vi "Plugin.Create.vi"(5 "Debug Flags":refnum<class "Debug Flags.lvclass">, 7 "transceiver count":i32, 8 "error in (no error)":errorcluster, 9 "component classes":refnum<class>[](array[class]), 10 "Plugin Configuration":refnum<class "Plugin Configuration.lvclass">, 11 "Transfer Groups":refnum<class "Transfer Group.lvclass">[](array[class])) -> (0 "error out":errorcluster, 2 "Transceiver":refnum<class "Transceiver.lvclass">, 3 "Plugin out":refnum<class "Plugin.lvclass">)   [LabVIEW 2017, in "DSF Core.lvlib" / "Plugin.lvclass"]
uses:
  Plugin.lvclass
  Transfer/Transfer Group.lvclass
  Debug/Debug Flags.lvclass
  Shared/Classes/Plugin/Plugin Configuration.lvclass
  C:/Git/DSF/dsf core/Source/Shared/Classes/Configuration/Configuration.lvclass
  Transceiver/Transceiver.lvclass
  Shared/Classes/Configuration/Configuration.lvclass/Configuration.ctl
  Shared/Classes/Plugin/Plugin Configuration.lvclass/Plugin Configuration.ctl
  Plugin.lvclass/Plugin.ctl
  Timing/Timing.lvclass
  Shared/Classes/Configuration/Configuration.lvclass
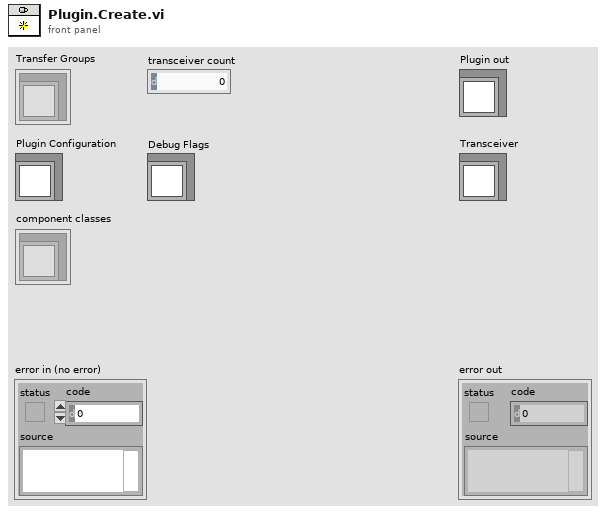
[diagram p1: front panel]
types:
  T1 = typedef "DSF Core.lvlib/DSF Timing Info.ctl" = cluster{"priority":u64, "decimation":u64, "offset":u64}
  T2 = typedef "DSF Core.lvlib/DSF Settings Info.ctl" = cluster{"key":string, "value":string}[]
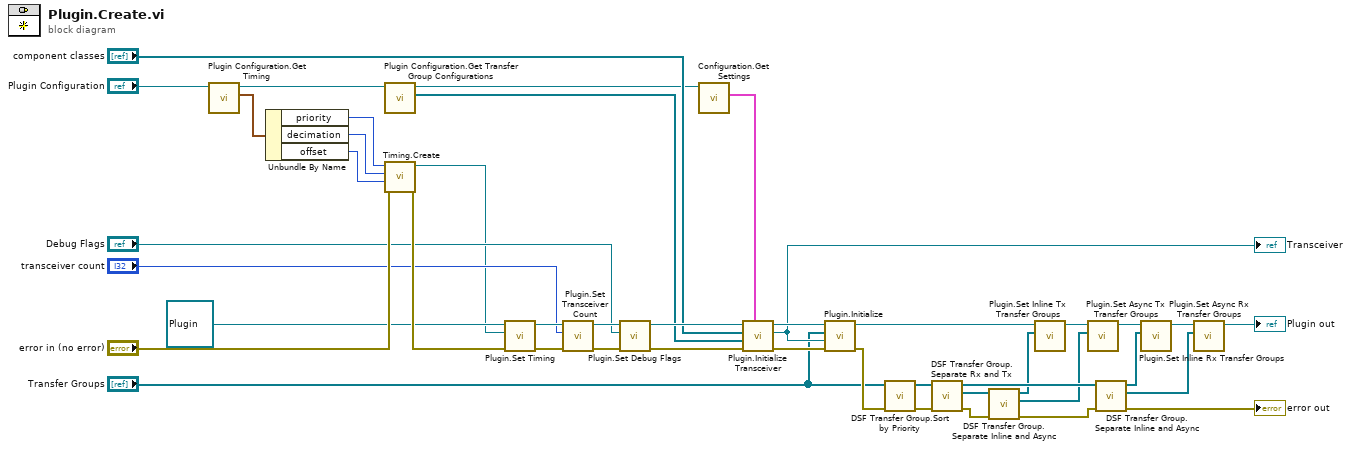
[diagram p0: block diagram]
diagram:
  n1 = call "Plugin Configuration.Get Timing.vi"("Plugin Configuration in"="Plugin Configuration") -> ("cycle timing"=w16:T1, "Plugin Configuration out"=w11:refnum<class "Plugin Configuration.lvclass">)  [unwired: 9 in]
  n2 = Unbundle By Name(w16) -> ("priority"=w13:u64, "decimation"=w14:u64, "offset"=w15:u64)
  n3 = call "Plugin Configuration.Get Transfer Group Configurations.vi"("Plugin Configuration in"=w11) -> ("Transfer Group Configurations"=w6:refnum<class "Transfer Group Configuration.lvclass">[], "Plugin Configuration out"=w2:refnum<class "Plugin Configuration.lvclass">)  [unwired: 9 in]
  n4 = call "Timing.Create.vi"("error in (no error)"="error in (no error)", "Offset"=w15, "Decimation"=w14, "Priority"=w13) -> ("error out"=w39:errorcluster, "Timing"=w10:refnum<class "Timing.lvclass">)  [unwired: 6 in]
  n5 = call "Plugin.Set Timing.vi"("Timing"=w10, "Plugin in"=refnum<class "Plugin.lvclass"> refnum) -> ("Plugin out"=w36:refnum<class "Plugin.lvclass">)  [unwired: 9 in]
  n6 = call "Plugin.Set Transceiver Count.vi"("transceiver count"="transceiver count", "Plugin in"=w36) -> ("Plugin out"=w23:refnum<class "Plugin.lvclass">)  [unwired: 9 in]
  n7 = call "Plugin.Set Debug Flags.vi"("Debug Flags"="Debug Flags", "Plugin in"=w23) -> ("Plugin out"=w9:refnum<class "Plugin.lvclass">)  [unwired: 9 in]
  n8 = call "Configuration.Get Settings.vi"("Configuration in"=w2) -> ("settings"=w1:T2)  [unwired: 9 in, 1 out]
  n9 = call "Plugin.Initialize Transceiver.vi"("transceiver settings"=w1, "error in (no error)"=w39, "Transfer Groups Configurations"=w6, "component classes"="component classes", "Plugin in"=w9) -> ("error out"=w4:errorcluster, "Transceiver"=w5:refnum<class "Transceiver.lvclass">, "Plugin out"=w8:refnum<class "Plugin.lvclass">)  [unwired: 4 in]
  "Transceiver" <- w5
  n10 = call "Plugin.Initialize.vi"("error in (no error)"=w4, "Transceiver"=w5, "Transfer Groups"="Transfer Groups", "Plugin in"=w8) -> ("error out"=w19:errorcluster, "Plugin out"=w21:refnum<class "Plugin.lvclass">)  [unwired: 6 in]
  n11 = call "DSF Transfer Group.Sort by Priority.vi"("error in (no error)"=w19, "Transfer Groups"="Transfer Groups") -> ("error out"=w38:errorcluster, "sorted Transfer Groups"=w37:refnum<class "Transfer Group.lvclass">[])  [unwired: 8 in]
  n12 = call "DSF Transfer Group.Separate Rx and Tx.vi"("error in (no error)"=w38, "Transfer Groups"=w37) -> ("error out"=w34:errorcluster, "Tx Transfer Groups"=w33:refnum<class "Transfer Group.lvclass">[], "Rx Transfer Groups"=w32:refnum<class "Transfer Group.lvclass">[])  [unwired: 7 in]
  n13 = call "DSF Transfer Group.Separate Inline and Async.vi"("error in (no error)"=w34, "Transfer Groups"=w33) -> ("error out"=w31:errorcluster, "Async Transfer Groups"=w29:refnum<class "Transfer Group.lvclass">[], "Inline Transfer Groups"=w30:refnum<class "Transfer Group.lvclass">[])  [unwired: 7 in]
  n14 = call "Plugin.Set Inline Tx Transfer Groups.vi"("Inline Tx Transfer Groups"=w30, "Plugin in"=w21) -> ("Plugin out"=w28:refnum<class "Plugin.lvclass">)  [unwired: 9 in]
  n15 = call "Plugin.Set Async Tx Transfer Groups.vi"("Async Tx Transfer Groups"=w29, "Plugin in"=w28) -> ("Plugin out"=w26:refnum<class "Plugin.lvclass">)  [unwired: 9 in]
  n16 = call "DSF Transfer Group.Separate Inline and Async.vi"("error in (no error)"=w31, "Transfer Groups"=w32) -> ("error out"=→"error out":errorcluster, "Async Transfer Groups"=w24:refnum<class "Transfer Group.lvclass">[], "Inline Transfer Groups"=w27:refnum<class "Transfer Group.lvclass">[])  [unwired: 7 in]
  n17 = call "Plugin.Set Inline Rx Transfer Groups.vi"("Inline Rx Transfer Groups"=w27, "Plugin in"=w26) -> ("Plugin out"=w25:refnum<class "Plugin.lvclass">)  [unwired: 9 in]
  n18 = call "Plugin.Set Async Rx Transfer Groups.vi"("Async Rx Transfer Groups"=w24, "Plugin in"=w25) -> ("Plugin out"=→"Plugin out":refnum<class "Plugin.lvclass">)  [unwired: 9 in]
